vi "Untitled 1.vi"() -> ()   [LabVIEW 2018]
panel:
  in  "push master":bool
  out "Slide 2":u8(slide) scale=0.0..100.0
  in  "Slide":dbl(slide) scale=0.0..10.0
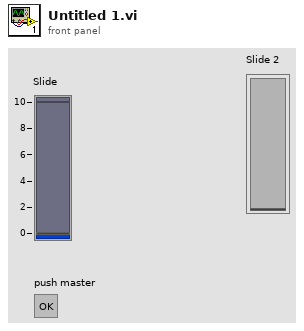
[diagram p1: front panel]
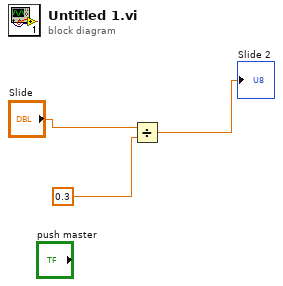
[diagram p0: block diagram]
diagram:
  n1 = Divide(x="Slide", y=0.3) -> (x/y=→"Slide 2":dbl)
